vi "select offset array.vi"(2 "MCL offset scanning range (V)":T2={"Min X"=5.0, "Max X"=10.0, "Min Y"=5.0, "Max Y"=10.0, "Scan increment"=5.0}, 3 "Offset File step size":dbl, 4 "Multi-MCL offset array":T1(array[cluster]), 5 "Trap position array":dbl[](array[numeric])) -> (0 "Out offsets":dbl[](array[numeric]), 1 "In range?":bool)   [LabVIEW 2014]
uses:
  <vilib>/imath/engines/lvmath2/RunTimeEngine/RunTimeType/NIMS_RunTimeType_From StrictType (excl LVString).vi
  <instcachedir>/0/NIMS_RunTimeType_From StrictType (excl LVString)_15A5391EEA9C4AACB9955AC755B83D29.lvgen/NIMS_RunTimeType_From StrictType (excl LVString)_15A5391EEA9C4AACB9955AC755B83D29_010.vi
  <vilib>/imath/engines/lvmath2/RunTimeEngine/Struct/NIMS_StructSetField.vi
  <vilib>/imath/engines/lvmath2/RunTimeEngine/IndexRead/NIMS M(S,S).vi
  <instcachedir>/0/NIMS M(S,S)_AC51E74150A542F7991B9634C66F3096.lvgen/NIMS M(S,S)_AC51E74150A542F7991B9634C66F3096_002.vi
  <vilib>/imath/engines/lvmath2/RunTimeEngine/Struct/NIMS_StructGetField.vi
  <vilib>/imath/engines/lvmath2/RunTimeEngine/RunTimeType/NIMS_RunTimeType_To Numeric.vi
  <instcachedir>/0/NIMS_RunTimeType_To Numeric_CEDD3DBADEB64FB59CD8C53099B6B149.lvgen/NIMS_RunTimeType_To Numeric_CEDD3DBADEB64FB59CD8C53099B6B149_004.vi
  <vilib>/imath/engines/lvmath2/RunTimeEngine/ArithmeticOperatorToken/NIMS_ArithmeticOperator_plus.vi
  <instcachedir>/0/NIMS_ArithmeticOperator_plus_48D6EAACA5D645B09F7EC9C016C2DEA8.lvgen/NIMS_ArithmeticOperator_plus_48D6EAACA5D645B09F7EC9C016C2DEA8_001.vi
  <instcachedir>/0/NIMS_RunTimeType_From StrictType (excl LVString)_15A5391EEA9C4AACB9955AC755B83D29.lvgen/NIMS_RunTimeType_From StrictType (excl LVString)_15A5391EEA9C4AACB9955AC755B83D29_007.vi
  <vilib>/imath/engines/lvmath2/RunTimeEngine/ErrorHandling/NIMS_Create Error From Enums.vi
  <instcachedir>/0/NIMS_ArithmeticOperator_plus_48D6EAACA5D645B09F7EC9C016C2DEA8.lvgen/NIMS_ArithmeticOperator_plus_48D6EAACA5D645B09F7EC9C016C2DEA8_004.vi
  <vilib>/imathl/engines/lvmath/Functions/Error Handling/Create Error.vi
  <instcachedir>/0/NIMS_RunTimeType_To Numeric_CEDD3DBADEB64FB59CD8C53099B6B149.lvgen/NIMS_RunTimeType_To Numeric_CEDD3DBADEB64FB59CD8C53099B6B149_002.vi
  <vilib>/imath/engines/lvmath2/RunTimeEngine/IndexRead/NIMS V(S).vi
  <instcachedir>/0/NIMS V(S)_0488751826AF41519A22953C041130DC.lvgen/NIMS V(S)_0488751826AF41519A22953C041130DC_003.vi
  <vilib>/imath/engines/lvmath2/RunTimeEngine/IndexReplace/NIMS V(S)=S.vi
  <instcachedir>/0/NIMS V(S)=S_2D52C4EC15D8415E870AEE69FB516CCA.lvgen/NIMS V(S)=S_2D52C4EC15D8415E870AEE69FB516CCA_001.vi
  <vilib>/imath/engines/lvmath2/RunTimeEngine/NodeEndStatement/NIMS_NodeEndStatement_Output.vi
  <instcachedir>/0/NIMS_NodeEndStatement_Output_53EC0D466D134D7ABD903AC30B43404B.lvgen/NIMS_NodeEndStatement_Output_53EC0D466D134D7ABD903AC30B43404B_000.vi
  <vilib>/imath/engines/lvmath2/RunTimeEngine/ErrorHandling/NIMS_Finalize Error.vi
panel:
  in  "error in (no error)":errorcluster
  out "error out":errorcluster
  out "Array":i32[](array[numeric])
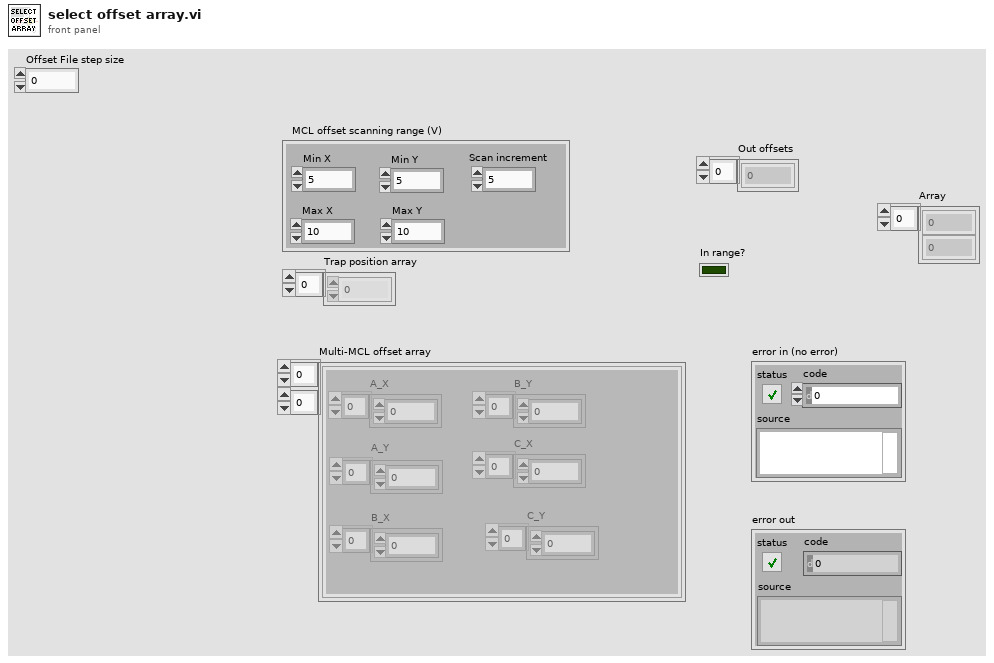
[diagram p1: front panel]
types:
  T1 = cluster{"A_X":dbl[], "A_Y":dbl[], "B_X":dbl[], "B_Y":dbl[], "C_X":dbl[], "C_Y":dbl[]}[][]
  T2 = cluster{"Min X":dbl, "Max X":dbl, "Min Y":dbl, "Max Y":dbl, "Scan increment":dbl}
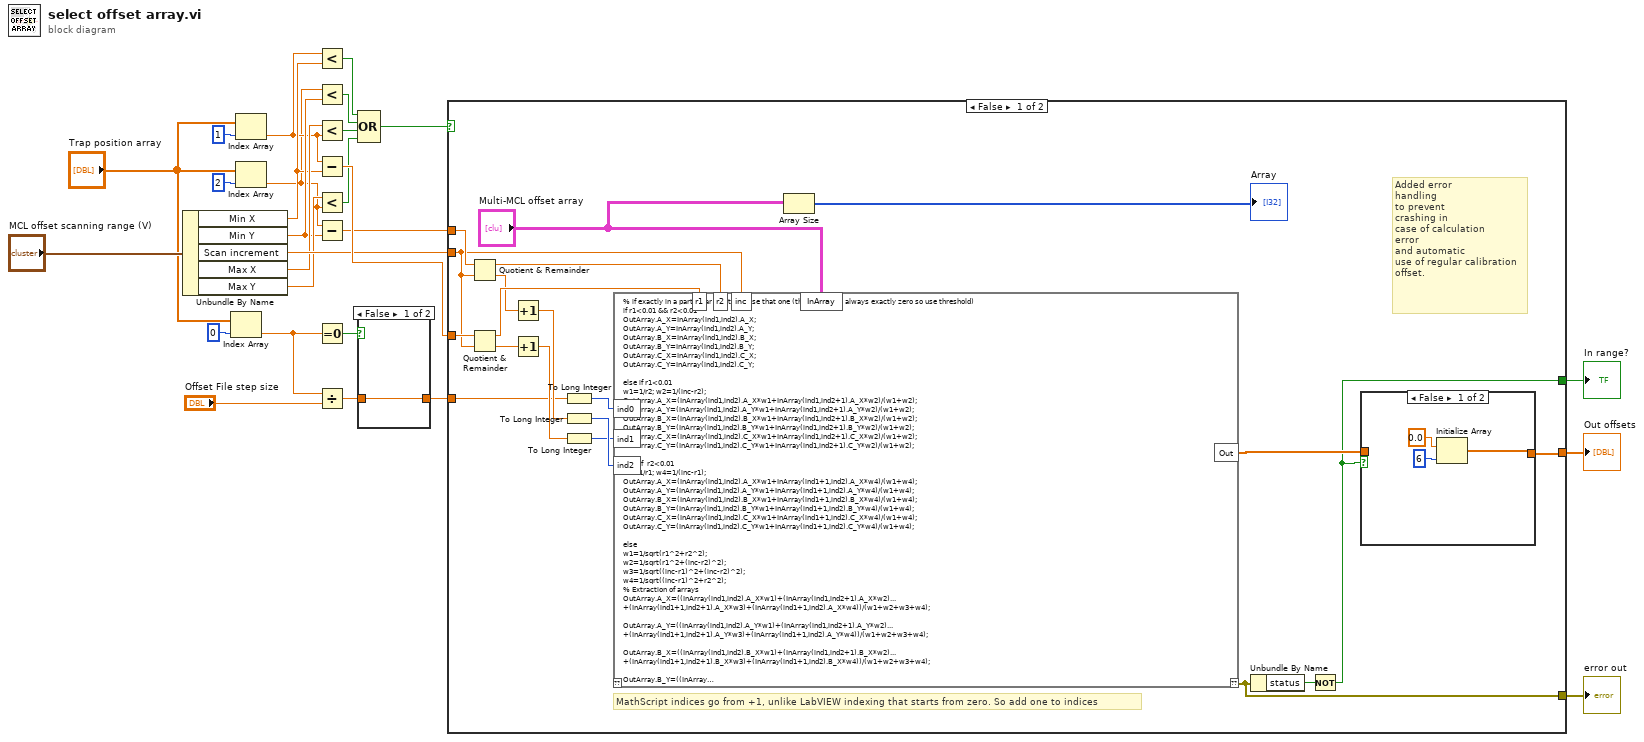
[diagram p0: block diagram]
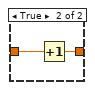
[diagram p2: hidden frame]
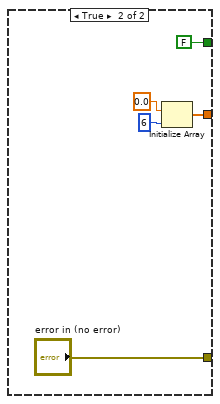
[diagram p4: hidden frame]
diagram:
  n1 = Unbundle By Name("MCL offset scanning range (V)") -> ("Min X"=w14:dbl, "Min Y"=w15:dbl, "Scan increment"=w22:dbl, "Max X"=w17:dbl, "Max Y"=w16:dbl)
  n2 = Index Array(array="Trap position array", index=0) -> (element=w5:dbl)
  n3 = Index Array(array="Trap position array", index=1) -> (element=w13:dbl)
  n4 = Index Array(array="Trap position array", index=2) -> (element=w12:dbl)
  n5 = Less?(x=w13, y=w14) -> (x < y?=w11:bool)
  n6 = Less?(x=w12, y=w15) -> (x < y?=w10:bool)
  n7 = Less?(x=w17, y=w13) -> (x < y?=w9:bool)
  n8 = Subtract(x=w13, y=w14) -> (x-y=w27:dbl)
  n9 = Less?(x=w16, y=w12) -> (x < y?=w8:bool)
  n10 = Subtract(x=w12, y=w15) -> (x-y=w26:dbl)
  n11 = Equal To 0?(x=w5) -> (x = 0?=w4:bool)
  n12 = Divide(x=w5, y="Offset File step size") -> (x/y=w3:dbl)
  n13 = Compound Arithmetic op=OR(w11, w10, w9, w8) -> (w7:bool)
  n14 = case shown="False" w4 {
    tunnel: w3 -> [w28 w30]
    tunnel: [w28 w29] -> w2
    frame False {
    }
    frame True {
      n15 = Increment(x=w30) -> (x+1=w29:dbl)
    }
  }
  n16 = case shown="False" w7 {
    tunnel: w27 -> [w50 _]
    tunnel: w26 -> [w49 _]
    tunnel: w22 -> [w46 _]
    tunnel: [w32 w1789] -> w18
    tunnel: w2 -> [w37 _]
    tunnel: [w31 FALSE] -> w6
    tunnel: [w35 "error in (no error)"] -> w1
    frame False {
      # "Added error\nhandling \nto prevent\ncrashing in\ncase of calculation\nerror \nand automatic \nuse of regular calibration\noffset."
      # "MathScript indices go from +1, unlike LabVIEW indexing that starts from zero. So add one to indices"
      n17 = Quotient & Remainder(x=w49, y=w46) -> (x-y*floor(x/y)=w47:dbl, floor(x/y)=w44:dbl)
      n18 = Quotient & Remainder(x=w50, y=w46) -> (x-y*floor(x/y)=w48:dbl, floor(x/y)=w45:dbl)
      n19 = Increment(x=w44) -> (x+1=w41:dbl)
      n20 = Increment(x=w45) -> (x+1=w39:dbl)
      n21 = To Long Integer(number=w37) -> (32bit integer=w36:i32)
      n22 = To Long Integer(number=w41) -> (32bit integer=w40:i32)
      n23 = To Long Integer(number=w39) -> (32bit integer=w38:i32)
      n24 = mathscript code="% if exactly in a particular point just use that one (the r's are not always exactly zero so use threshold)\nif r1<0.01 && r2<0.01\nOutArray.A_X=InArray(ind1,ind2).A_X;\nOutArray.A_Y=InArray(ind1,ind2).A_Y;\nOutArray.B_X=InArray(ind1,ind2).B_X;\nOutArray.B_Y=InArray(ind1,ind2).B_Y;\nOutArray.C_X=InArray(ind1,ind2).C_X;\nOutArray.C_Y=InArray(ind1,ind2).C_Y;\n\nelse if r1<0.01\nw1=1/r2; w2=1/(inc-r2);\nOutArray.A_X=(InArray(ind1,ind2).A_X*w1+InArray(ind1,ind2+1).A_X*w2)/(w1+w2);\nOutArray.A_Y=(InArray(ind1,ind2).A_Y*w1+InArray(ind1,ind2+1).A_Y*w2)/(w1+w2);\nOutArray.B_X=(InArray(ind1,ind2).B_X*w1+InArray(ind1,ind2+1).B_X*w2)/(w1+w2);\nOutArray.B_Y=(InArray(ind1,ind2).B_Y*w1+InArray(ind1,ind2+1).B_Y*w2)/(w1+w2);\nOutArray.C_X=(InArray(ind1,ind2).C_X*w1+InArray(ind1,ind2+1).C_X*w2)/(w1+w2);\nOutArray.C_Y=(InArray(ind1,ind2).C_Y*w1+InArray(ind1,ind2+1).C_Y*w2)/(w1+w2);\n\nelse if  r2<0.01\nw1=1/r1; w4=1/(inc-r1);\nOutArray.A_X=(InArray(ind1,ind2).A_X*w1+InArray(ind1+1,ind2).A_X*w4)/(w1+w4);\nOutArray.A_Y=(InArray(ind1,ind2).A_Y*w1+InArray(ind1+1,ind2).A_Y*w4)/(w1+w4);\nOutArray.B_X=(InArray(ind1,ind2).B_X*w1+InArray(ind1+1,ind2).B_X*w4)/(w1+w4);\nOutArray.B_Y=(InArray(ind1,ind2).B_Y*w1+InArray(ind1+1,ind2).B_Y*w4)/(w1+w4);\nOutArray.C_X=(InArray(ind1,ind2).C_X*w1+InArray(ind1+1,ind2).C_X*w4)/(w1+w4);\nOutArray.C_Y=(InArray(ind1,ind2).C_Y*w1+InArray(ind1+1,ind2).C_Y*w4)/(w1+w4);\n\nelse \nw1=1/sqrt(r1^2+r2^2);\nw2=1/sqrt(r1^2+(inc-r2)^2);\nw3=1/sqrt((inc-r1)^2+(inc-r2)^2);\nw4=1/sqrt((inc-r1)^2+r2^2);\n% Extraction of arrays\nOutArray.A_X=((InArray(ind1,ind2).A_X*w1)+(InArray(ind1,ind2+1).A_X*w2)...\n+(InArray(ind1+1,ind2+1).A_X*w3)+(InArray(ind1+1,ind2).A_X*w4))/(w1+w2+w3+w4);\n\nOutArray.A_Y=((InArray(ind1,ind2).A_Y*w1)+(InArray(ind1,ind2+1).A_Y*w2)...\n+(InArray(ind1+1,ind2+1).A_Y*w3)+(InArray(ind1+1,ind2).A_Y*w4))/(w1+w2+w3+w4);\n\nOutArray.B_X=((InArray(ind1,ind2).B_X*w1)+(InArray(ind1,ind2+1).B_X*w2)...\n+(InArray(ind1+1,ind2+1).B_X*w3)+(InArray(ind1+1,ind2).B_X*w4))/(w1+w2+w3+w4);\n\nOutArray.B_Y=((InArray(ind1,ind2).B_Y*w1)+(InArray(ind1,ind2+1).B_Y*w2)...\n+(InArray(ind1+1,ind2+1).B_Y*w3)+(InArray(ind1+1,ind2).B_Y*w4))/(w1+w2+w3+w4);\n\nOutArray.C_X=((InArray(ind1,ind2).C_X*w1)+(InArray(ind1,ind2+1).C_X*w2)...\n+(InArray(ind1+1,ind2+1).C_X*w3)+(InArray(ind1+1,ind2).C_X*w4))/(w1+w2+w3+w4);\n\nOutArray.C_Y=((InArray(ind1,ind2).C_Y*w1)+(InArray(ind1,ind2+1).C_Y*w2)...\n+(InArray(ind1+1,ind2+1).C_Y*w3)+(InArray(ind1+1,ind2).C_Y*w4))/(w1+w2+w3+w4);\n\nend\nend\nend\n\nOut(1)=OutArray.A_X(ind0); Out(2)=OutArray.A_Y(ind0); Out(3)=OutArray.B_X(ind0); \nOut(4)=OutArray.B_Y(ind0); Out(5)=OutArray.C_X(ind0); Out(6)=OutArray.C_Y(ind0);"("r1"=w48, "r2"=w47, "inc"=w46, "InArray"="Multi-MCL offset array", "ind1"=w38, "ind2"=w40, "ind0"=w36) -> ("??"=w35:errorcluster, "Out"=w33:cdb[])  [unwired: 1 in]
      n25 = Array Size(array="Multi-MCL offset array") -> (size(s)=→"Array":i32[])
      n26 = Unbundle By Name(w35) -> ("status"=w34:bool)
      n27 = Not(x=w34) -> (.not. x?=w31:bool)
      n28 = case shown="False" w31 {
        tunnel: [w51 w54] -> w32
        tunnel: w33 -> [_ w54]
        frame False {
          n29 = Initialize Array(0.0, 6) -> (w51:dbl[])
        }
        frame True {
        }
      }
    }
    frame True {
      n30 = Initialize Array(0.0, 6) -> (w1789:dbl[])
    }
  }
  "Out offsets" <- w18
  "In range?" <- w6
  "error out" <- w1
